vi "Flatten Value.vi"(8 "error in (no error)":errorcluster, 11 "Boolean in":refnum<class "Timestamp.lvclass">) -> (0 "error out":errorcluster, 2 "Value":string, 3 "Boolean out":refnum<class "Timestamp.lvclass">)   [LabVIEW 2019, in "Timestamp.lvclass"]
uses:
  <vilib>/gpm_packages/@cs/data-type-serializer/source/Timestamp/Timestamp.lvclass
  <vilib>/gpm_packages/@cs/data-type-serializer/source/Timestamp/Timestamp.lvclass/Timestamp.ctl
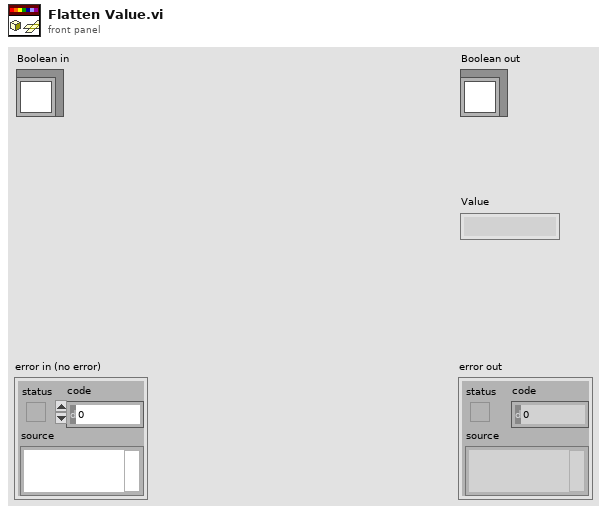
[diagram p1: front panel]
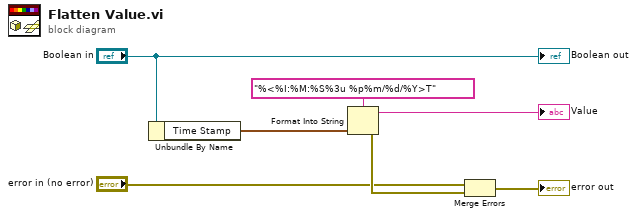
[diagram p0: block diagram]
diagram:
  n1 = Unbundle By Name("Boolean in") -> ("Time Stamp"=w5:timestamp)
  n2 = Format Into String(format string="%<%I:%M:%S%3u %p%m/%d/%Y>T", w5) -> (resulting string=→"Value":string, error out=w3:errorcluster)  [unwired: 2 in]
  n3 = Merge Errors("error in (no error)", w3) -> (→"error out":errorcluster)
  "Boolean out" <- "Boolean in"
